vi "Fetch Acquired Data (U64).vi"(5 "FIFO Type":T1, 7 "Timeout (s)":i32=5, 8 "error out":errorcluster, 9 "Swap?":bool, 10 "Samples":i32=-1, 11 "FPGA Reference In":refnum<k20>) -> (0 "error out":errorcluster, 2 "Data":u64[](array[numeric]), 3 "FPGA Reference Out":refnum<k20>, 4 "Elements Remaining":u32)   [LabVIEW 2012, in "FlexRIO Host Library (User).lvlib"]
uses:
  <userlib>/FlexRIO Host Library/FlexRIO Host Library (User).lvlib
  <userlib>/FlexRIO Host Library/FlexRIO Host API/Acquire/FIFO Type.ctl
  <vilib>/Utility/error.llb/Error Cluster From Error Code.vi
  <vilib>/rvi/errors/niLvFpgaAdjustHostInterfaceError.vi
  <vilib>/rvi/interface/nirviMethod/nirviMethod.xnode
  <vilib>/rvi/errors/niLvFpgaMergeErrorWithErrorCode.vi
  <vilib>/FPGAPlugInAG/Dynamic/niLvFpga_ReadFifo_Dynamic.vi
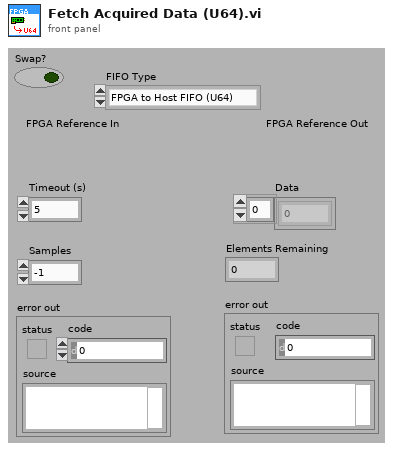
[diagram p1: front panel]
types:
  T1 = typedef "FIFO Type.ctl" = enum16{"FPGA to Host FIFO (U64)", "Generic", "FPGA to Host FIFO (U32)"}
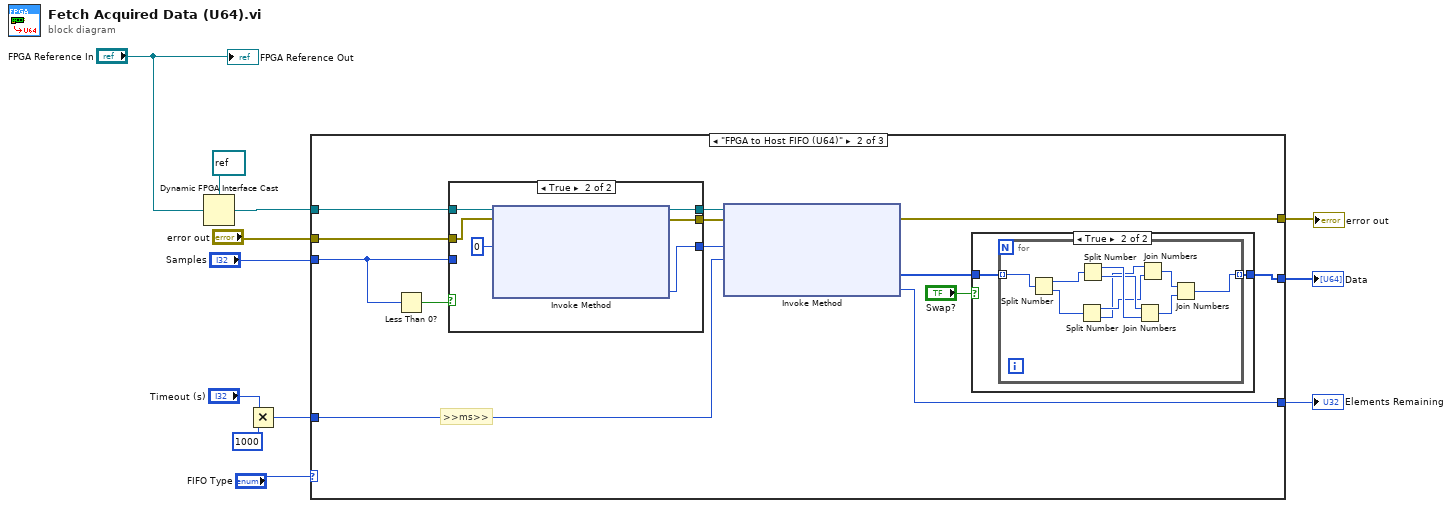
[diagram p0: block diagram]
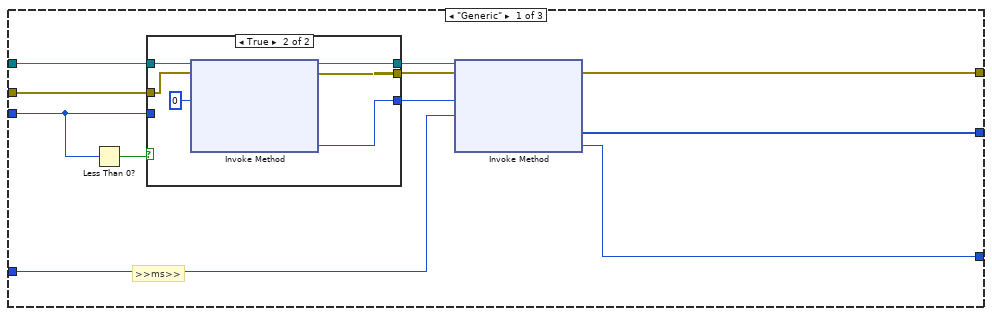
[diagram p2: hidden frame]
diagram:
  n1 = Dynamic FPGA Interface Cast(Session In=refnum<k20> refnum ("Type"), Type="FPGA Reference In") -> (Session Out=w10:refnum<k20>)
  n2 = Multiply(x="Timeout (s)", y=1000) -> (x*y=w3:i32)
  n3 = case shown="\"FPGA to Host FIFO (U64)\"" "FIFO Type" {
    tunnel: [w19 w34 _] -> w12
    tunnel: w10 -> [w18 w41 _]
    tunnel: [w17 w40 w68] -> w9
    tunnel: [w16 w39 _] -> w8
    tunnel: "error out" -> [w14 w38 w68]
    tunnel: "Samples" -> [w13 w37 _]
    tunnel: w3 -> [w15 w36 _]
    frame "Generic" {
      # ">>ms>>"
      n4 = Less Than 0?(x=w13) -> (x < 0?=w23:bool)
      n5 = case shown="True" w23 {
        tunnel: w18 -> [w26 w32]
        tunnel: w14 -> [w25 w31]
        tunnel: [w26 w30] -> w22
        tunnel: [w25 w29] -> w21
        tunnel: [w24 w28] -> w20
        tunnel: w13 -> [w24 _]
        frame False {
        }
        frame True {
          n6 = xnode "Invoke Method"("FPGA VI Reference In"=w32, "error in"=w31, "Number of Elements"=u32 0) -> ("FPGA VI Reference Out"=w30:refnum<k20>, "error out"=w29:errorcluster, "Elements Remaining"=w28:u32)  [unwired: 1 in, 1 out]
        }
      }
      n7 = xnode "Invoke Method"("FPGA VI Reference In"=w22, "error in"=w21, "Number of Elements"=w20, "Timeout (ms)"=w15) -> ("error out"=w17:errorcluster, "Data"=w19:u64[], "Elements Remaining"=w16:u32)  [unwired: 1 out]
    }
    frame "FPGA to Host FIFO (U64)" {
      # ">>ms>>"
      n8 = Less Than 0?(x=w37) -> (x < 0?=w45:bool)
      n9 = case shown="True" w45 {
        tunnel: w41 -> [w61 w67]
        tunnel: w38 -> [w60 w66]
        tunnel: [w61 w65] -> w44
        tunnel: [w60 w64] -> w43
        tunnel: [w59 w63] -> w42
        tunnel: w37 -> [w59 _]
        frame False {
        }
        frame True {
          n10 = xnode "Invoke Method"("FPGA VI Reference In"=w67, "error in"=w66, "Number of Elements"=u32 0) -> ("FPGA VI Reference Out"=w65:refnum<k20>, "error out"=w64:errorcluster, "Elements Remaining"=w63:u32)  [unwired: 1 in, 1 out]
        }
      }
      n11 = xnode "Invoke Method"("FPGA VI Reference In"=w44, "error in"=w43, "Number of Elements"=w42, "Timeout (ms)"=w36) -> ("error out"=w40:errorcluster, "Data"=w35:u64[], "Elements Remaining"=w39:u32)  [unwired: 1 out]
      n12 = case shown="True" "Swap?" {
        tunnel: w35 -> [w46 w48]
        tunnel: [w46 w47] -> w34
        frame False {
        }
        frame True {
          n13 = for {
            tunnel: w48 -> [w58] mode=indexing
            tunnel: [w49] -> w47 mode=indexing
            n14 = Split Number(x=w58) -> (hi(x)=w56:u32, lo(x)=w57:u32)
            n15 = Split Number(x=w57) -> (hi(x)=w53:u16, lo(x)=w52:u16)
            n16 = Split Number(x=w56) -> (hi(x)=w55:u16, lo(x)=w54:u16)
            n17 = Join Numbers(hi=w54, lo=w55) -> ((hi.lo)=w50:u32)
            n18 = Join Numbers(hi=w52, lo=w53) -> ((hi.lo)=w51:u32)
            n19 = Join Numbers(hi=w51, lo=w50) -> ((hi.lo)=w49:u64)
          }
        }
      }
    }
    frame "FPGA to Host FIFO (U32)" {
    }
  }
  "Data" <- w12
  "error out" <- w9
  "Elements Remaining" <- w8
  "FPGA Reference Out" <- "FPGA Reference In"
